vi "Oscilloscope_Dual Ch_Separate storage_with name.vi"() -> ()   [LabVIEW 2024]
uses:
  <vilib>/DAQmx/read.llb/DAQmx Read (Analog 1D Wfm NChan NSamp).vi
  <vilib>/DAQmx/create/channels.llb/DAQmx Create Channel (AI-Voltage-Basic).vi
  <vilib>/DAQmx/configure/timing.llb/DAQmx Timing (Sample Clock).vi
  <vilib>/DAQmx/miscellaneous.llb/DAQmx Fill In Error Info.vi
  <vilib>/ptbypt/NI_PtbyPt.lvlib
panel:
  in  "physical channels":tag="cDAQ2Mod1/ai0, cDAQ2Mod1/ai3"
  in  "File Name":string
  in  "Amplitude, Ch2":dbl(knob)=2.0815012654367786 scale=0.0..10.0
  in  "Time Window, Ch2":dbl(knob)=0.044976272347247236 scale=1e-08..0.1
  in  "Channel 2":bool=TRUE
  out "Left":dynamicdata(graph)=[{"t0"=timestamp(3806599236.6321588 s since 1904-01-01), "dt"=4.999999999999579e-07, "Y"=array[202167 elements], "attributes"=variant("NI_ChannelName"=variant(string "cDAQ2Mod1/ai1"), "NI_UnitDescription"=variant(string "Volts"))}]
  in  "Amplitude, Ch1":dbl(knob)=3.274182299184287 scale=0.0..10.0
  in  "Record":bool
  in  "Time Window, Ch1":dbl(knob)=0.04438102924292822 scale=1e-05..0.1
  out "Right":dynamicdata(graph)=[{"t0"=timestamp(3806599236.6321588 s since 1904-01-01), "dt"=4.999999999999579e-07, "Y"=array[202167 elements], "attributes"=variant("NI_ChannelName"=variant(string "cDAQ2Mod1/ai0"), "NI_UnitDescription"=variant(string "Volts"))}]
  in  "stop":bool
  in  "Channel 1":bool=TRUE
  in  "Folder to save file to":path=path "A:/Source Localization/Material Evaluation paper/Dataset/Microphone Characterization/Clean Source"
  in  "Sample Rate":dbl=200000.0 format="%0.2f"
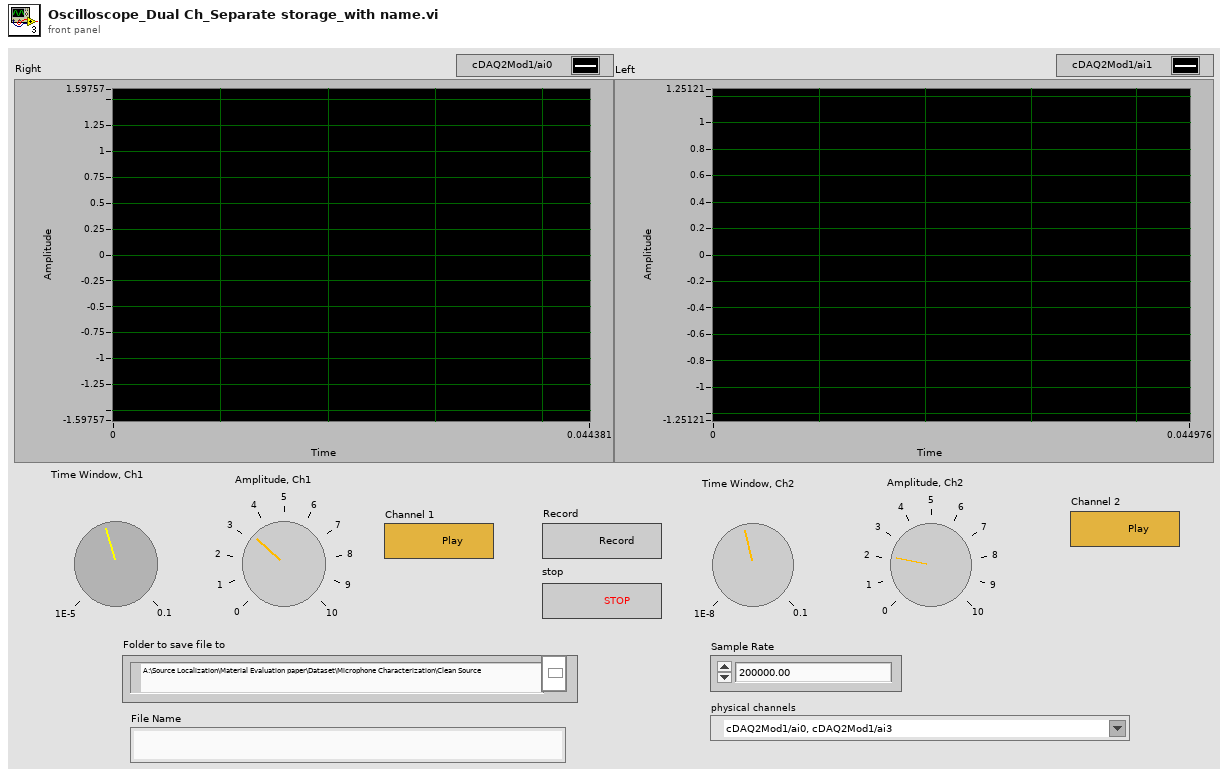
[diagram p1: front panel]
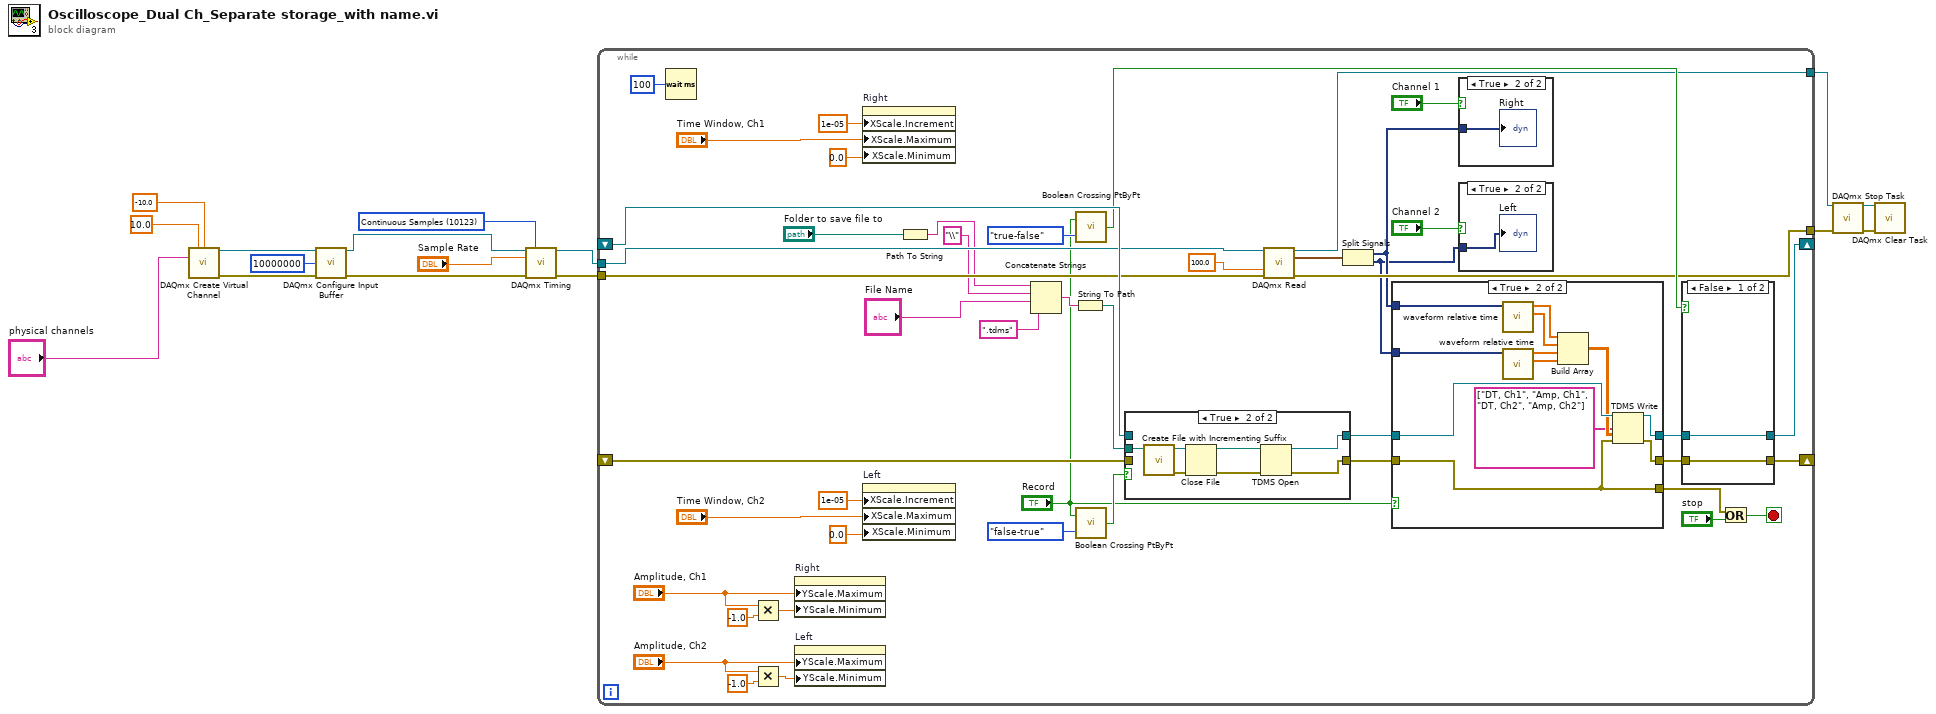
[diagram p0: block diagram]
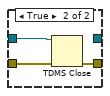
[diagram p4: hidden frame]
diagram:
  w4 = 10123 items=["Finite Samples"=10178, "Continuous Samples"=10123, "Hardware Timed Single Point"=12522] ("sample mode")
  n1 = call-poly <vilib>:"DAQmx Create Virtual Channel.vi"("maximum value"=10.0, "minimum value"=-10.0, "physical channels"="physical channels") -> ("task out"=w16:refnum<k21>, "error out"=w15:errorcluster)  [unwired: 11 in]
  n2 = call <vilib>:"DAQmx Configure Input Buffer.vi"("task/channels in"=w16, "buffer size (in samples per channel)"=u32 10000000, "error in"=w15) -> ("task out"=w13:refnum<k21>, "error out"=w12:errorcluster)  [unwired: 11 in]
  n3 = call-poly <vilib>:"DAQmx Timing.vi"("task/channels in"=w13, "sample mode"=w4, "rate"="Sample Rate", "error in"=w12) -> ("task out"=w10:refnum<k21>, "error out"=w9:errorcluster)  [unwired: 10 in]
  n4 = while {
    shift-right: [w55] -> _
    shift-left: _ -> [w60]
    tunnel: w10 -> [w54]
    tunnel: w9 -> [w53]
    tunnel: [w50] -> w8
    tunnel: [w49] -> w7
    shift-right: [w40] -> _
    shift-left: _ -> [w33]
    stop <- w51 stop-if-true
    n5 = Wait (ms)(milliseconds to wait=u32 100) -> ()  [unwired: 1 out]
    n6 = Multiply(x="Amplitude, Ch1", y=-1.0) -> (x*y=w30:dbl)
    n7 = Multiply(x="Amplitude, Ch2", y=-1.0) -> (x*y=w23:dbl)
    n8 = property on="Right" class="WFGraph (strict)"("YScale.Maximum"="Amplitude, Ch1", "YScale.Minimum"=w30) -> ()  [unwired: 2 in, 2 out]
    n9 = property on="Left" class="WFGraph (strict)"("YScale.Maximum"="Amplitude, Ch2", "YScale.Minimum"=w23) -> ()  [unwired: 2 in, 2 out]
    n10 = property on="Right" class="WFGraph (strict)"("XScale.Increment"=1e-05 ("X Scale.Range:Increment"), "XScale.Maximum"="Time Window, Ch1", "XScale.Minimum"=0.0 ("X Scale.Range:Minimum")) -> ()  [unwired: 2 in, 2 out]
    n11 = property on="Left" class="WFGraph (strict)"("XScale.Increment"=1e-05 ("X Scale.Range:Increment"), "XScale.Maximum"="Time Window, Ch2", "XScale.Minimum"=0.0 ("X Scale.Range:Minimum")) -> ()  [unwired: 2 in, 2 out]
    n12 = Path To String(path="Folder to save file to") -> (string=w46:string)
    n13 = Concatenate Strings(w46, "\\" ("string"), "File Name", ".tdms" ("string")) -> (w45:string)
    n14 = String To Path(string=w45) -> (path=w44:path)
    n15 = call <vilib>:"Boolean Crossing PtByPt.vi"("direction"=enum16{"either", "false-true", "true-false"}."true-false", "input"="Record") -> ("crossing"=w58:bool)  [unwired: 1 in]
    n16 = call <vilib>:"Boolean Crossing PtByPt.vi"("direction"=enum16{"either", "false-true", "true-false"}."false-true", "input"="Record") -> ("crossing"=w56:bool)  [unwired: 1 in]
    n17 = case shown="True" w56 {
      tunnel: [w85 w92] -> w62
      tunnel: w60 -> [w85 _]
      tunnel: w44 -> [_ w90]
      tunnel: [w84 w91] -> w39
      tunnel: w33 -> [w84 _]
      frame False {
      }
      frame True {
        n18 = call <vilib>:"Create File with Incrementing Suffix.vi"("file path"=w90) -> ("error out"=w88:errorcluster, "refnum out"=w89:refnum<file>)  [unwired: 8 in, 1 out]
        n19 = Close File(refnum=w89, error in=w88) -> (path=w86:path, error out=w87:errorcluster)
        n20 = TDMS Open(8:w87, 11:w86) -> (0:w91:errorcluster, 3:w92:refnum<k34>)  [unwired: 5 in]
      }
    }
    n21 = call-poly <vilib>:"DAQmx Read.vi"("task/channels in"=w54, "timeout"=100.0, "error in"=w53) -> ("task out"=w50:refnum<k21>, "data"=w27:waveform(dbl)[], "error out"=w49:errorcluster)  [unwired: 10 in]
    n22 = Split Signals(w27) -> (w20:dynamicdata, w19:dynamicdata)  [unwired: 2 in]
    n23 = case shown="True" "Record" {
      tunnel: w62 -> [w71 w83]
      tunnel: [w71 w82] -> w61
      tunnel: w39 -> [w70 w77]
      tunnel: [w70 w78] -> w38
      tunnel: [w70 w77] -> w34
      tunnel: w20 -> [_ w75]
      tunnel: w19 -> [_ w74]
      frame False {
      }
      frame True {
        n24 = call "waveform relative time.vi"("signal in"=w75) -> ("Y"=w80:dbl[], "Relative Time"=w81:dbl[])  [unwired: 7 in, 2 out]
        n25 = call "waveform relative time.vi"("signal in"=w74) -> ("Y"=w72:dbl[], "Relative Time"=w73:dbl[])  [unwired: 7 in, 2 out]
        n26 = Build Array(w81, w80, w73, w72) -> (w79:dbl[][])
        n27 = TDMS Write(0:w83, 7:string[] ["DT, Ch1", "Amp, Ch1", "DT, Ch2", "Amp, Ch2"] ("channel name(s) in (Untitled)"), 9:w79, 11:w77) -> (4:w82:refnum<k34>, 15:w78:errorcluster)  [unwired: 2 in, 2 out]
      }
    }
    n28 = case shown="True" "Channel 1" {
      tunnel: w20 -> [_ w64]
      frame False {
      }
      frame True {
        "Right" <- w64
      }
    }
    n29 = case shown="True" "Channel 2" {
      tunnel: w19 -> [_ w63]
      frame False {
      }
      frame True {
        "Left" <- w63
      }
    }
    n30 = case shown="False" w58 {
      tunnel: w61 -> [w66 w69]
      tunnel: [w66 _] -> w55
      tunnel: [w65 w68] -> w40
      tunnel: w38 -> [w65 w67]
      frame False {
      }
      frame True {
        n31 = TDMS Close(8:w67, 11:w69) -> (0:w68:errorcluster)  [unwired: 1 out]
      }
    }
    n32 = Or(x=w34, y="stop") -> (x .or. y?=w51:bool)
  }
  n33 = call <vilib>:"DAQmx Stop Task.vi"("task/channels in"=w8, "error in"=w7) -> ("task out"=w6:refnum<k21>, "error out"=w5:errorcluster)  [unwired: 12 in]
  n34 = call <vilib>:"DAQmx Clear Task.vi"("task in"=w6, "error in"=w5) -> ()  [unwired: 13 in, 1 out]
